vi "Comunicacion serial.vi"(0 "VISA resource name":refnum<visa-resource-name>="COM1", 1 "baud rate":u32=9600, 2 "data bits":u16=8 min=5 max=8 step=1, 3 "parity":u16(ring) items=["None", "Odd", "Even", "Mark", "Space"], 4 "stop bits":u16(ring)=10 items=["1.0"=10, "1.5"=15, "2.0"=20], 7 "flow control":u16(ring) items=["None"=0, "XON/XOFF"=1, "RTS/CTS"=2, "DTR/DSR"=4]) -> ()   [LabVIEW 2010]
doc: "The Basic Serial Read and Write example performs a Serial Port Read, a Serial Port Write, or a combination of these actions. The user selects the actions (read or write) on the front panel. If both are selected, the VI will write the data first, read data, and then close the VISA session that is opened to the port. This VI will wait until the specified number of bytes is received at the port. Only the number of bytes specified will be read.\n\nINSTRUCTIONS:\n1) Select the serial resource and configuration parameters (baud rate, data bits, parity, stop bits, flow control).\n2) Select the operations to be performed. \n3) Connect the serial port to your device. If no device is available, perform a loopback test by doing one of the following. Short pins 2 and 3 on a RS-232 cable or short pin 4 to pin 8 and pin 5 to pin 9 on a RS-485/422 cable. \n4) Run the VI to see the data read. (The \"read string\" will match the \"string to write\" if a loopback test was performed.)\n\nNote: The parameters set for the serial port must match the parameters of the connected instrument or device. In this example, the bytes to read parameter specifies the number of bytes that the serial port reads. If there were more bytes at the port than the number specified in bytes to read, those bytes would not be read. Also, if you specify to read more bytes than the number of bytes actually read, you might receive a timeout error message.\n\nOn the block diagram, the Configure Serial Port VI sets the configuration parameters. The front panel displays the controls used to configure the basic parameters, such as baud rate, data bits, and parity. Constants configure the other parameters the user probably does not need set. After the VISA Configure Serial Port VI opens the VISA session and configures the port, the VI passes the VISA resource name to other VIs that perform operations on that VISA resource. The VISA Write function sends a command to the serial device and the VISA Read function returns data based on the command. The VISA Close function then closes the reference to the serial device. It is important to close the reference; otherwise communication through with that port through protocols other than VISA might not be possible."
uses:
  <vilib>/Instr/_visa.llb/VISA Configure Serial Port (Instr).vi
panel:
  out "CORRECCION \nLATERAL FINAL \n(mils)":dbl
  in  "RONZA MILS":dbl(knob) scale=800.0..1600.0
  in  "Derecha/Izquierda":bool
  in  "DIRECCION DEL VIENTO":dbl
  in  "CORRECCION DEL VIENTO\n LATERAL(mils)":dbl
  in  "INTENSIDAD VIENTO (m/s)":dbl
  in  "MARCACION (Grad)":dbl
  in  "CARGA":dbl
  in  "RANGO CORREGIDO":dbl
  in  "MILS":dbl
  in  "ELEVACION MILS":dbl(slide) scale=800.0..1511.0
  in  "ELEVACION GRADOS":dbl(slide) scale=44.8..84.6
  in  "RONZA GRADOS":dbl(slide) scale=45.0..90.0
  out "Numeric":i32
  out "Angulo":dbl[](graph)
  in  "correccion de temp. (m)":dbl
  in  "RANGO (m)":dbl
  out "Temp Terrmocupla":i32
  out "read buffer":string
  in  "stop":bool
  out "Temperatura":i32[](graph)
  out "Termocupla":dbl(slide) scale=0.0..150.0 scale format="%#_6f"
  in  "delay before read (ms)":u32=500
  # "COM SERIAL"
  # "CORRECCION EN ELEVACION"
  # "DATOS INICIALES"
  # "SOLUCION DE TIRO (ELEVACION)"
  # "CONTROL DE RONZA"
  # "DATOS INICIALES"
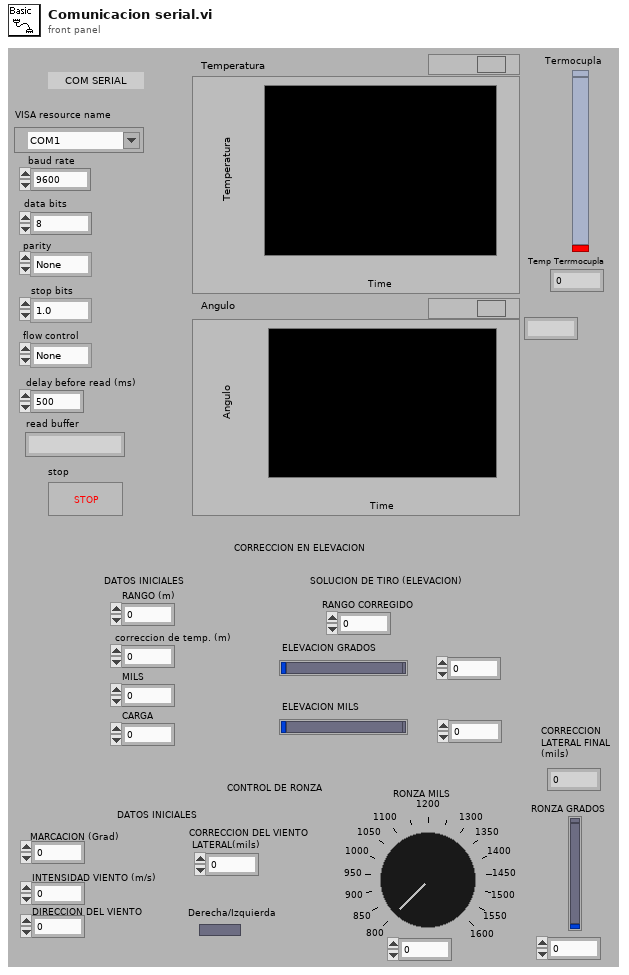
[diagram p1: front panel]
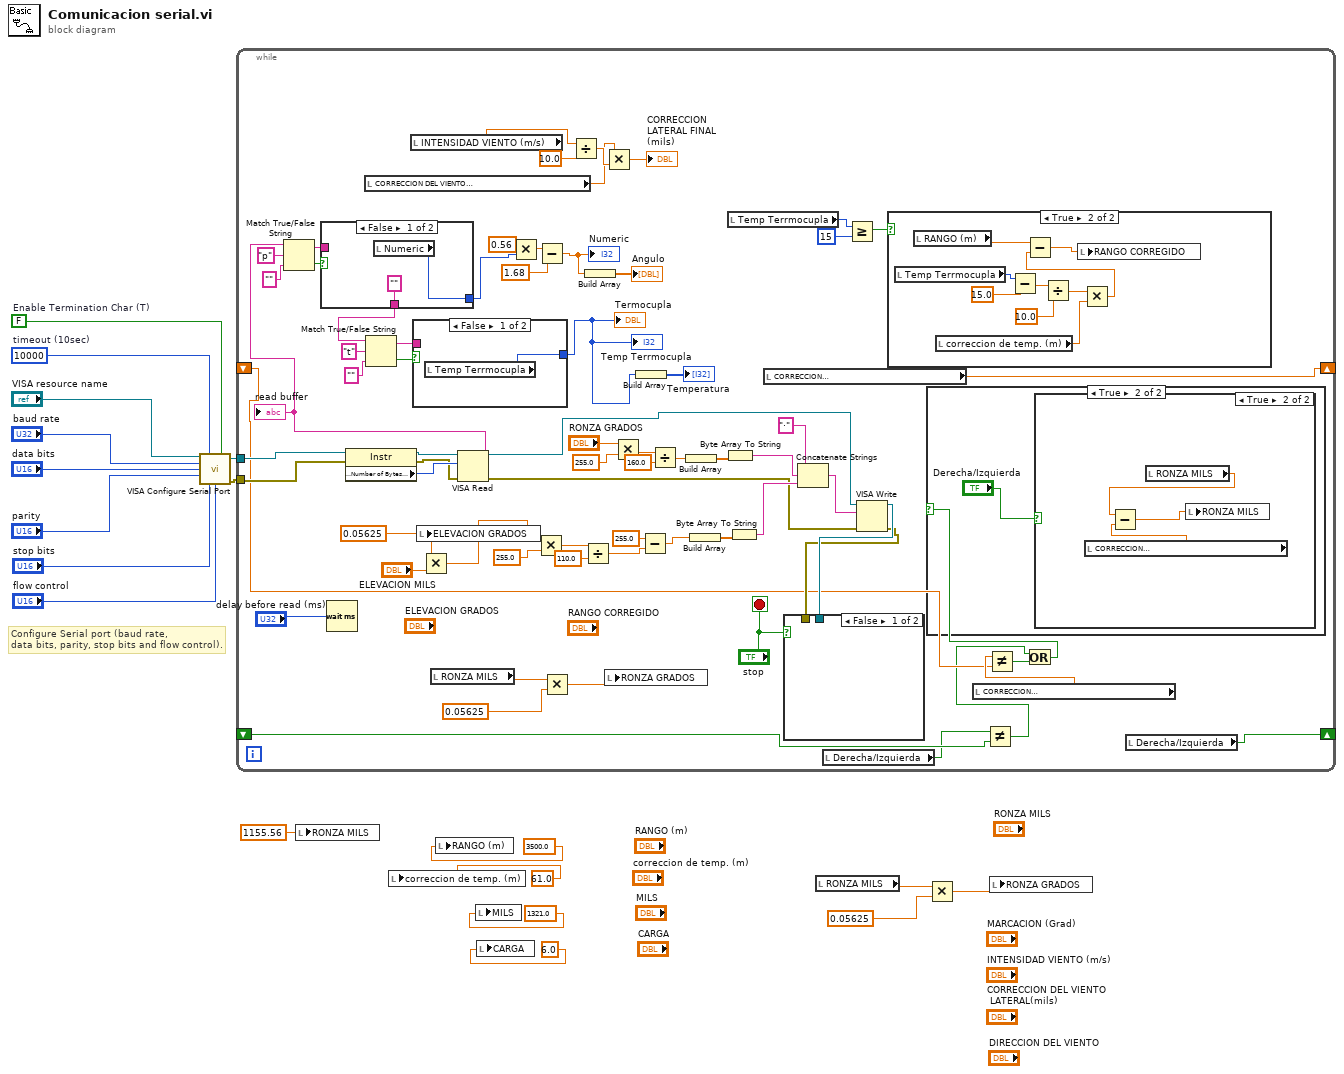
[diagram p0: block diagram]
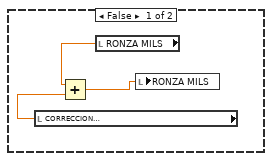
[diagram p3: hidden frame]
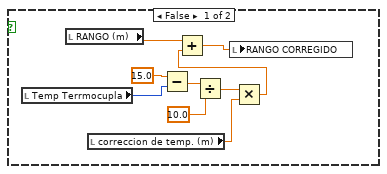
[diagram p4: hidden frame]
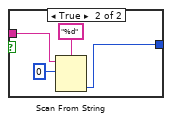
[diagram p5: hidden frame]
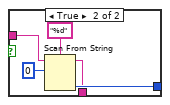
[diagram p6: hidden frame]
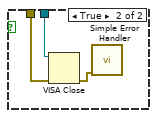
[diagram p7: hidden frame]
diagram:
  w13 = FALSE  # Enable Termination Char (T)
  w14 = u32 10000  # timeout (10sec)
  # "Configure Serial port (baud rate,\ndata bits, parity, stop bits and flow control)."
  n1 = call-poly "VISA Configure Serial Port"("VISA resource name"="VISA resource name", "timeout (10sec)"=w14, "Enable Termination\nChar (T)"=w13, "baud rate (9600)"="baud rate", "data bits (8)"="data bits", "parity (0:none)"="parity", "stop bits (10: 1 bit)"="stop bits", "flow control (0:none)"="flow control") -> ("VISA resource name out"=w16:refnum<visa-resource-name>, "error out"=w9:errorcluster)  [unwired: 6 in]
  n2 = while {
    tunnel: w9 -> [w86]
    tunnel: w16 -> [w82]
    shift-right: [w35] -> _
    shift-left: _ -> [w33]
    shift-right: [w31] -> _
    shift-left: _ -> [w28]
    stop <- "stop" stop-if-true
    n3 = Wait (ms)(milliseconds to wait="delay before read (ms)") -> ()  [unwired: 1 out]
    n4 = property class="Instr"(reference=w82, error in=w86) -> (reference out=w85:refnum<visa-resource-name>, error out=w83:errorcluster, "Serial Settings:Number of Bytes at Serial Port"=w84:u32)
    n5 = local read "CORRECCION DEL VIENTO\n LATERAL(mils)"() -> (w20:dbl)
    n6 = local read "INTENSIDAD VIENTO (m/s)"() -> (w22:dbl)
    n7 = Multiply(x=0.05625, y="ELEVACION MILS") -> (x*y=w39:dbl)
    n8 = local write "ELEVACION GRADOS"(w39) -> ()
    n9 = local read "RONZA MILS"() -> (w25:dbl)
    n10 = VISA Read(VISA resource name=w85, byte count=w84, error in (no error)=w83) -> (VISA resource name out=w65:refnum<visa-resource-name>, read buffer=w76:string, error out=w64:errorcluster)  [unwired: 1 out]
    "read buffer" <- w76
    n11 = Match True/False String(2:"" ("false string"), 3:"p" ("true string"), 4:w76) -> (0:w79:bool, 1:w78:string)
    n12 = case shown="False" w79 {
      tunnel: w78 -> [_ w122]
      tunnel: [w119 w121] -> w46
      tunnel: ["" w120] -> w53
      frame False {
        n13 = local read "Numeric"() -> (w119:i32)
      }
      frame True {
        n14 = Scan From String(format string="%d", input string=w122, initial scan location=u32 0) -> (remaining string=w120:string, output 1=w121:i32)  [unwired: 2 in, 2 out]
      }
    }
    n15 = Match True/False String(2:"" ("false string"), 3:"t" ("true string"), 4:w53) -> (0:w52:bool, 1:w51:string)
    n16 = case shown="False" w52 {
      tunnel: w51 -> [_ w115]
      tunnel: [w113 w114] -> w49
      frame False {
        n17 = local read "Temp Terrmocupla"() -> (w113:i32)
      }
      frame True {
        n18 = Scan From String(format string="%d", input string=w115, initial scan location=u32 0) -> (output 1=w114:i32)  [unwired: 2 in, 3 out]
      }
    }
    "Termocupla" <- w49
    "Temp Terrmocupla" <- w49
    n19 = Multiply(x=0.56, y=w46) -> (x*y=w45:dbl)
    n20 = Multiply(x=w39, y=255.0) -> (x*y=w60:dbl)
    n21 = Subtract(x=w45, y=1.68) -> (x-y=w43:dbl)
    "Numeric" <- w43
    n22 = Multiply(x=w25, y=0.05625 ("x")) -> (x*y=w26:dbl)
    n23 = Divide(x=w22, y=10.0) -> (x/y=w21:dbl)
    n24 = Divide(x=w60, y=110.0) -> (x/y=w58:dbl)
    n25 = Build Array(w43) -> (→"Angulo":dbl[])
    n26 = Multiply(x=w20, y=w21) -> (x*y=→"CORRECCION \nLATERAL FINAL \n(mils)":dbl)
    n27 = local write "RONZA GRADOS"(w26) -> ()
    n28 = Multiply(x="RONZA GRADOS", y=255.0) -> (x*y=w73:dbl)
    n29 = Build Array(w49) -> (→"Temperatura":i32[])
    n30 = Subtract(x=255.0, y=w58) -> (x-y=w57:dbl)
    n31 = Divide(x=w73, y=160.0) -> (x/y=w69:dbl)
    n32 = Build Array(w69) -> (w71:dbl[])
    n33 = Build Array(w57) -> (w56:dbl[])
    n34 = Byte Array To String(unsigned byte array=w71) -> (string=w67:string)
    n35 = local read "Temp Terrmocupla"() -> (w38:i32)
    n36 = Byte Array To String(unsigned byte array=w56) -> (string=w68:string)
    n37 = local read "CORRECCION \nLATERAL FINAL \n(mils)"() -> (w35:dbl)
    n38 = Concatenate Strings("·" ("string"), w67, w68) -> (w66:string)
    n39 = local read "Derecha/Izquierda"() -> (w27:bool)
    n40 = Greater Or Equal?(x=w38, y=15) -> (x >= y?=w36:bool)
    n41 = VISA Write(VISA resource name=w65, write buffer=w66, error in (no error)=w64) -> (VISA resource name out=w63:refnum<visa-resource-name>, error out=w62:errorcluster)  [unwired: 1 out]
    n42 = case shown="False" "stop" {
      tunnel: w63 -> [_ w126]
      tunnel: w62 -> [_ w125]
      frame False {
      }
      frame True {
        n43 = VISA Close(VISA resource name=w126, error in (no error)=w125) -> (error out=w127:errorcluster)
        n44 = call <vilib>:"Simple Error Handler.vi"("error in (no error)"=w127) -> ()  [unwired: 4 in, 5 out]
      }
    }
    n45 = case shown="True" w36 {
      frame False {
        n46 = local read "Temp Terrmocupla"() -> (w96:i32)
        n47 = local read "RANGO (m)"() -> (w103:dbl)
        n48 = local read "correccion de temp. (m)"() -> (w99:dbl)
        n49 = Subtract(x=15.0 ("y"), y=w96) -> (x-y=w102:dbl)
        n50 = Divide(x=w102, y=10.0) -> (x/y=w100:dbl)
        n51 = Multiply(x=w100, y=w99) -> (x*y=w98:dbl)
        n52 = Add(x=w103, y=w98) -> (x+y=w95:dbl)
        n53 = local write "RANGO CORREGIDO"(w95) -> ()
      }
      frame True {
        n54 = local read "Temp Terrmocupla"() -> (w110:i32)
        n55 = local read "RANGO (m)"() -> (w112:dbl)
        n56 = local read "correccion de temp. (m)"() -> (w106:dbl)
        n57 = Subtract(x=w110, y=15.0) -> (x-y=w109:dbl)
        n58 = Divide(x=w109, y=10.0) -> (x/y=w107:dbl)
        n59 = Multiply(x=w107, y=w106) -> (x*y=w105:dbl)
        n60 = Subtract(x=w112, y=w105) -> (x-y=w104:dbl)
        n61 = local write "RANGO CORREGIDO"(w104) -> ()
      }
    }
    n62 = local read "CORRECCION \nLATERAL FINAL \n(mils)"() -> (w34:dbl)
    n63 = Not Equal?(x=w27, y=w28) -> (x != y?=w30:bool)
    n64 = Not Equal?(x=w34, y=w33) -> (x != y?=w32:bool)
    n65 = Or(x=w30, y=w32) -> (x .or. y?=w29:bool)
    n66 = case shown="True" w29 {
      frame False {
      }
      frame True {
        n67 = case shown="True" "Derecha/Izquierda" {
          frame False {
            n68 = local read "CORRECCION \nLATERAL FINAL \n(mils)"() -> (w90:dbl)
            n69 = local read "RONZA MILS"() -> (w91:dbl)
            n70 = Add(x=w91, y=w90) -> (x+y=w89:dbl)
            n71 = local write "RONZA MILS"(w89) -> ()
          }
          frame True {
            n72 = local read "CORRECCION \nLATERAL FINAL \n(mils)"() -> (w92:dbl)
            n73 = local read "RONZA MILS"() -> (w93:dbl)
            n74 = Subtract(x=w93, y=w92) -> (x-y=w94:dbl)
            n75 = local write "RONZA MILS"(w94) -> ()
          }
        }
      }
    }
    n76 = local read "Derecha/Izquierda"() -> (w31:bool)
  }
  n77 = local write "RONZA MILS"(1155.56 ("RONZA MILS")) -> ()
  n78 = local write "correccion de temp. (m)"(61.0 ("correccion de temp. (m)")) -> ()
  n79 = local write "RANGO (m)"(3500.0 ("RANGO (m)")) -> ()
  n80 = local write "MILS"(1321.0 ("MILS")) -> ()
  n81 = local write "CARGA"(6.0 ("CARGA")) -> ()
  n82 = local read "RONZA MILS"() -> (w4:dbl)
  n83 = Multiply(x=w4, y=0.05625 ("x")) -> (x*y=w2:dbl)
  n84 = local write "RONZA GRADOS"(w2) -> ()
